vi "PH_Powermeter_BaseClass.set Energy.vi"(0 "VI in":refnum<vi>, 5 "error in (no error)":errorcluster) -> (14 "VI out":refnum<vi>, 19 "error out":errorcluster)   [LabVIEW 2014, in "PH_Powermeter_BaseClass.lvlib"]
uses:
  PH_Powermeter_BaseClass.lvlib
  CSlibraries-extern/DimLVEvent/LVDimInterface/LVDimInterface.lvlib
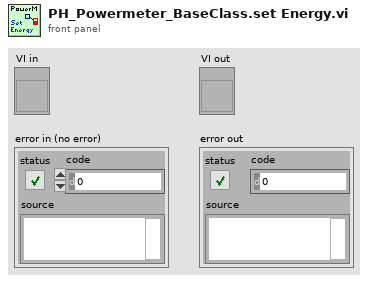
[diagram p1: front panel]
types:
  T1 = typedef "PH_Powermeter_BaseClass.lvlib/PH_Powermeter_BaseClass.i attribute.ctl" = cluster{"GUI References":T2, "Connection":T3, "Head Attributes":T5, "VISA resource":refnum<visa-resource-name>, "Energy":T6, "Service ID Energy":i32, "Wanted Settings":T7, "Current Settings":T7}
  T2 = typedef "PH_Powermeter_BaseClass.lvlib/PH_Powermeter_BaseClass.GUI Refs.ctl" = cluster{"Head Attributes":refnum<vi>, "Energy":refnum<vi>, "Connection":refnum<vi>, "VISA Resource":refnum<vi>, "Energy evolution":refnum<vi>, "Scaling Factor":refnum<vi>, "Range":refnum<vi>, "Wavelength":refnum<vi>, "Trigger Level":refnum<vi>, "Wanted Settings":refnum<vi>, "Current Settings":refnum<vi>}
  T3 = typedef "PH_Powermeter_BaseClass.lvlib/PH_Powermeter_BaseClass.Connection.ctl" = cluster{"failed checks":i8, "Timeout":bool, "Data read":string, "Failure":bool, "Error":bool, "State":T4}
  T4 = typedef "PH_Powermeter_BaseClass.lvlib/PH_Powermeter_BaseClass.State.ctl" = enum32{"off", "operating", "opened", "checked", "connected", "Sets to change", "running"}
  T5 = typedef "PH_Powermeter_BaseClass.lvlib/PH_Powermeter_BaseClass.Head Attributes.ctl" = cluster{"Instrument Type":string, "Head Version":string, "Head Name":string, "Serial Number":string, "Firmware":string, "Sensor Type":string, "MinimumRange":u32, "Maximum Range":u32, "Min Wavelength":i32, "Max Wavelength":i32}
  T6 = typedef "PH_Powermeter_BaseClass.lvlib/PH_Powermeter_BaseClass.Energy.ctl" = cluster{"current Value":dbl, "unscaled":dbl, "Scaling Factor":dbl}
  T7 = typedef "PH_Powermeter_BaseClass.lvlib/PH_gentec_BaseClass.Head Settings.ctl" = cluster{"Trigger Level":dbl, "Wavelength":u32, "Range":u32}
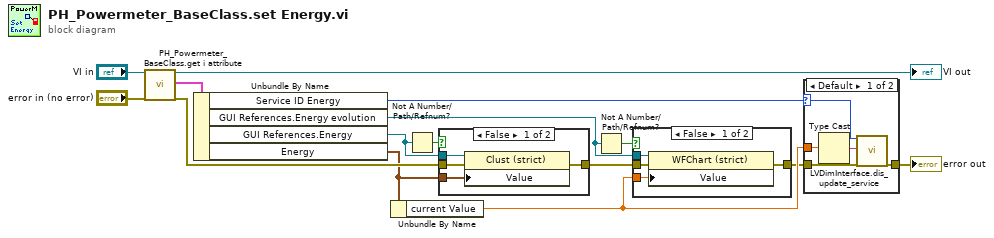
[diagram p0: block diagram]
diagram:
  n1 = call "PH_Powermeter_BaseClass.get i attribute.vi"("i ref in"="VI in", "error in (no error)"="error in (no error)") -> ("i ref out"=→"VI out":refnum<vi>, "i attribute"=w11:T1, "error out"=w15:errorcluster)  [unwired: 15 in]
  n2 = Unbundle By Name(w11) -> ("Service ID Energy"=w8:i32, "GUI References.Energy evolution"=w1:refnum<vi>, "GUI References.Energy"=w9:refnum<vi>, "Energy"=w6:T6)
  n3 = Unbundle By Name(w6) -> ("current Value"=w4:dbl)
  n4 = Not A Number/Path/Refnum?(number/path/refnum=w9) -> (NaN/Path/Refnum?=w10:bool)
  n5 = case shown="False" w10 {
    tunnel: w15 -> [w19 w20]
    tunnel: [w18 w20] -> w3
    tunnel: w9 -> [w17 _]
    tunnel: w6 -> [w16 _]
    frame False {
      n6 = property class="Clust (strict)"(reference=w17, error in=w19, "Value"=w16) -> (error out=w18:errorcluster)  [unwired: 1 out]
    }
    frame True {
    }
  }
  n7 = Not A Number/Path/Refnum?(number/path/refnum=w1) -> (NaN/Path/Refnum?=w5:bool)
  n8 = case shown="False" w5 {
    tunnel: w3 -> [w24 w25]
    tunnel: [w23 w25] -> w2
    tunnel: w1 -> [w22 _]
    tunnel: w4 -> [w21 _]
    frame False {
      n9 = property class="WFChart (strict)"(reference=w22, error in=w24, "Value"=w21) -> (error out=w23:errorcluster)  [unwired: 1 out]
    }
    frame True {
    }
  }
  n10 = case shown="Default" w8 {
    selector: w8 -> [w26 _]
    tunnel: w2 -> [w27 w31]
    tunnel: [w30 w31] -> w7
    tunnel: w4 -> [w29 _]
    frame Default {
      n11 = Type Cast(x=w29) -> (*(type *) &x=w28:string)  [unwired: 1 in]
      n12 = call "LVDimInterface.dis_update_service.vi"("my_serviceID"=w26, "data"=w28, "error in (no error)"=w27) -> ("error out"=w30:errorcluster)  [unwired: 14 in, 2 out]
    }
    frame -1 {
    }
  }
  "error out" <- w7
